vi "Refnum Initialize.vi"(8 "error in (no error)":errorcluster, 11 "XYGraphOverview in":refnum<class "XYGraphOverview.lvclass">) -> (0 "error out":errorcluster, 3 "XYGraphOverview out":refnum<class "XYGraphOverview.lvclass">)   [LabVIEW 2020, in "XYGraphOverview.lvlib" / "XYGraphOverview.lvclass"]
uses:
  XYGraphOverview.lvclass
  X Range Change User Event Data.ctl
  Caller User Event Data.ctl
  Command.ctl
  XYGraphOverview.lvclass/XYGraphOverview.ctl
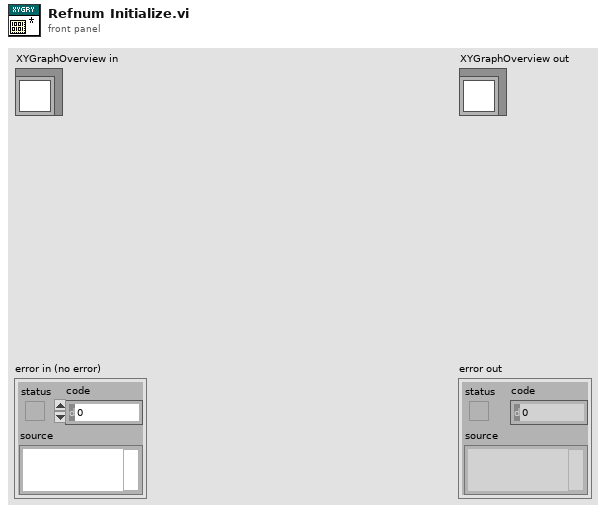
[diagram p1: front panel]
types:
  T1 = typedef "XYGraphOverview.lvlib/XYGraphOverview.lvclass/Caller User Event Data.ctl" = cluster{"Command":T2, "Data":variant}
  T2 = typedef "XYGraphOverview.lvlib/XYGraphOverview.lvclass/Command.ctl" = enum16{"Update Data", "Update Limit", "Zoom"}
  T3 = typedef "XYGraphOverview.lvlib/XYGraphOverview.lvclass/X Range Change User Event Data.ctl" = cluster{"Lower Range":dbl, "Upper Range":dbl, "All":bool}
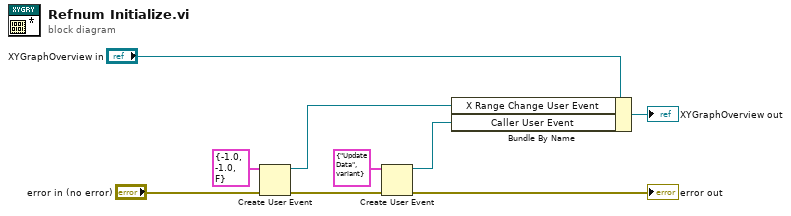
[diagram p0: block diagram]
diagram:
  n1 = Create User Event(user event datatype=T3 {"Lower Range"=-1.0, "Upper Range"=-1.0, "All"=FALSE} ("X Range Change User Event Data"), error in="error in (no error)") -> (user event=w4:refnum<user-event>, error out=w6:errorcluster)
  n2 = Create User Event(user event datatype=T1 {"Command"=enum."Update Data", "Data"=variant} ("Caller User Event"), error in=w6) -> (user event=w3:refnum<user-event>, error out=→"error out":errorcluster)
  n3 = Bundle By Name(cluster="XYGraphOverview in", "X Range Change User Event"=w4, "Caller User Event"=w3) -> (→"XYGraphOverview out":refnum<class "XYGraphOverview.lvclass">)
